vi "write_acq_time.vi"(8 "error in (no error)":errorcluster, 10 "acq_time":i32, 11 "detector in":refnum<class "detector.lvclass">) -> (0 "error out":errorcluster, 3 "detector out":refnum<class "detector.lvclass">)   [LabVIEW 2015, in "detector.lvclass"]
uses:
  detector.lvclass
  detector.lvclass/detector.ctl
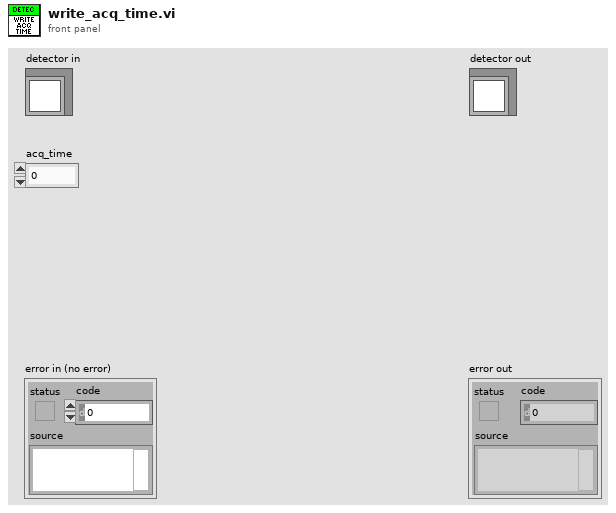
[diagram p1: front panel]
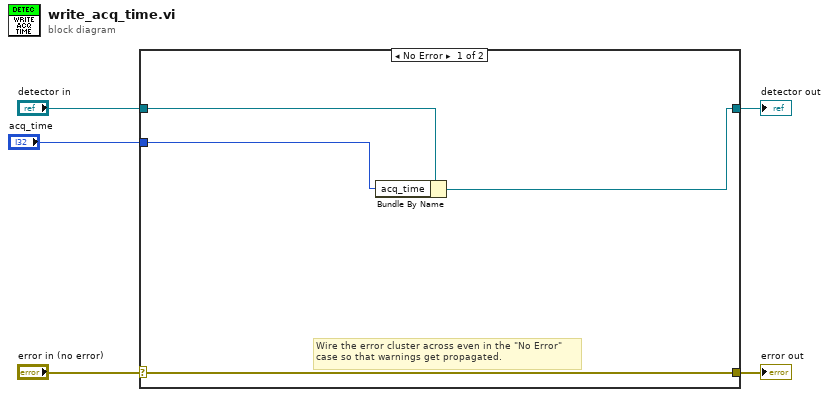
[diagram p0: block diagram]
diagram:
  n1 = case shown="No Error" "error in (no error)" {
    selector: "error in (no error)" -> [w9 w11]
    tunnel: [w9 w11] -> w4
    tunnel: [w6 w10] -> w2
    tunnel: "detector in" -> [w8 w10]
    tunnel: "acq_time" -> [w7 _]
    frame No Error {
      # "Wire the error cluster across even in the \"No Error\"\ncase so that warnings get propagated."
      n2 = Bundle By Name(cluster=w8, "acq_time"=w7) -> (w6:refnum<class "detector.lvclass">)
    }
    frame Error {
    }
  }
  "error out" <- w4
  "detector out" <- w2
